vi "Main.vi"(8 "error in":errorcluster, 11 "Maestro Acq in":refnum<class "Maestro Acq.lvclass">) -> (0 "error out":errorcluster, 3 "Maestro Acq out":refnum<class "Maestro Acq.lvclass">)   [LabVIEW 2021, in "Maestro Acq.lvclass"]
doc: "The Queued Message Handler of a Worker."
uses:
  Maestro Acq.lvclass
  C:/Program Files (x86)/National Instruments/LabVIEW 2021/vi.lib/addons/_Workers/Library/Classes/Worker/Worker.lvclass
  Acquisition State.ctl
  Initialization Data.ctl
  <vilib>/addons/_Workers/Library/Classes/Message Queue/Message Queue.lvclass
  Hardware Maestro Config.ctl
  Maestro Acq.lvclass/Maestro Acq.ctl
  <vilib>/addons/_Workers/Library/Classes/Message/Enqueue Message to Self v2 - Silent Mode.vi
  <vilib>/addons/_Workers/Library/Classes/Message/Enqueue Message to Self v2.vi
  <vilib>/addons/_Workers/Library/Classes/Message/Enqueue Message to Queue.vi
  <vilib>/addons/_Workers/Library/Classes/Message/Message.lvclass
  Maestro Control/Maestro Control.lvclass
  C:/Program Files (x86)/National Instruments/LabVIEW 2021/vi.lib/addons/_Workers/Library/Classes/Workers Object/Workers Object.lvclass
  C:/Users/flepetit/Desktop/Gentec-maestro-Labview/Workers/Maestro Acq/Maestro Acq.lvclass
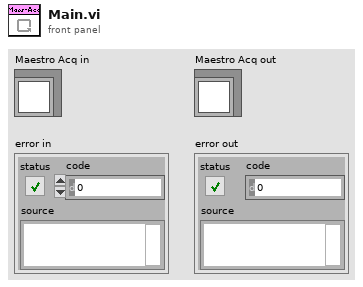
[diagram p1: front panel]
types:
  T1 = typedef "Maestro Acq.lvclass/Initialization Data.ctl" = cluster{"String":string, "Maestro Ctrl Queue":refnum<class "Message Queue.lvclass">, "Hardware Maestro Config":T2}
  T2 = typedef "Maestro Acq.lvclass/Hardware Maestro Config.ctl" = cluster{"Adress(ip)":string, "Port":i16}
  T3 = typedef "Maestro Acq.lvclass/Acquisition State.ctl" = enum16{"Idle", "Acquiring"}
  T4 = typedef "Workers.lvlib/Case Label.ctl" = string
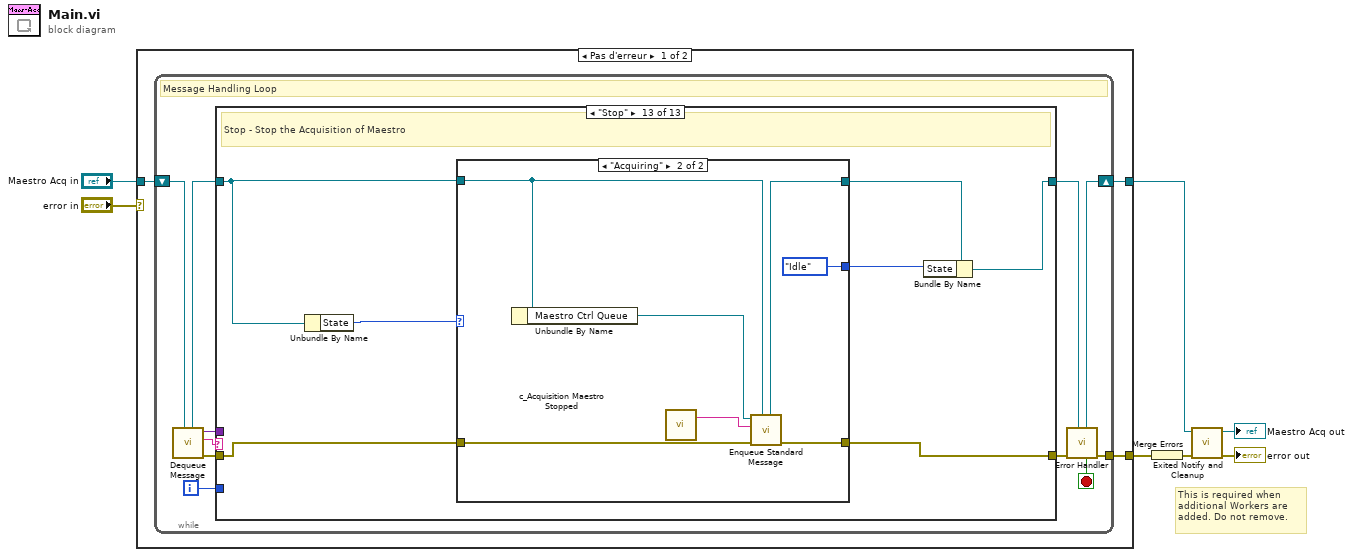
[diagram p0: block diagram]
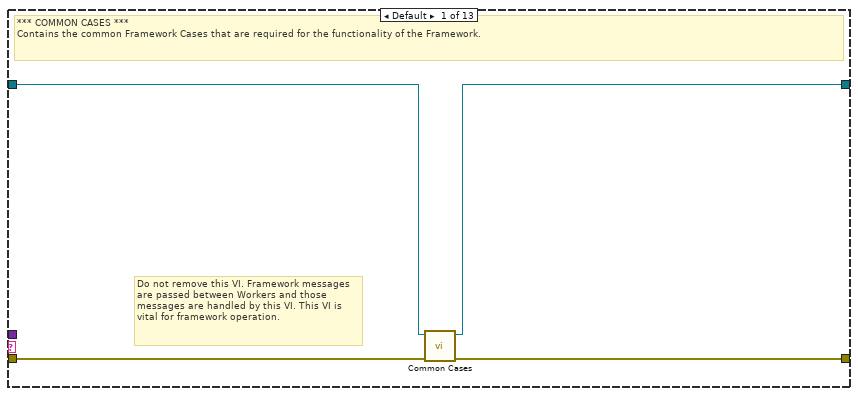
[diagram p2: hidden frame]
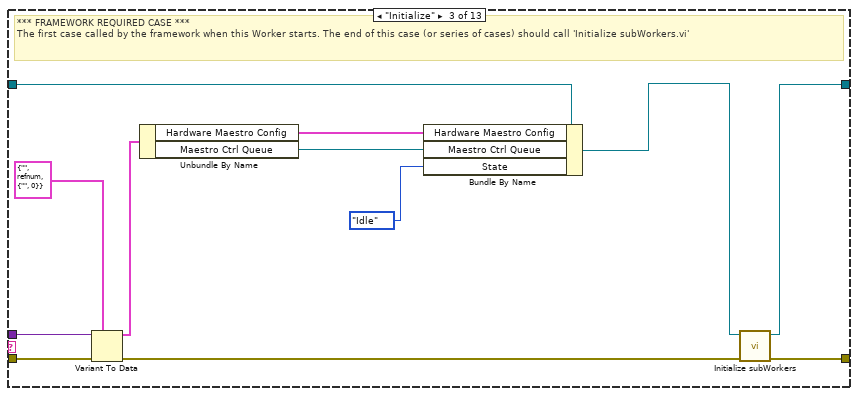
[diagram p4: hidden frame]
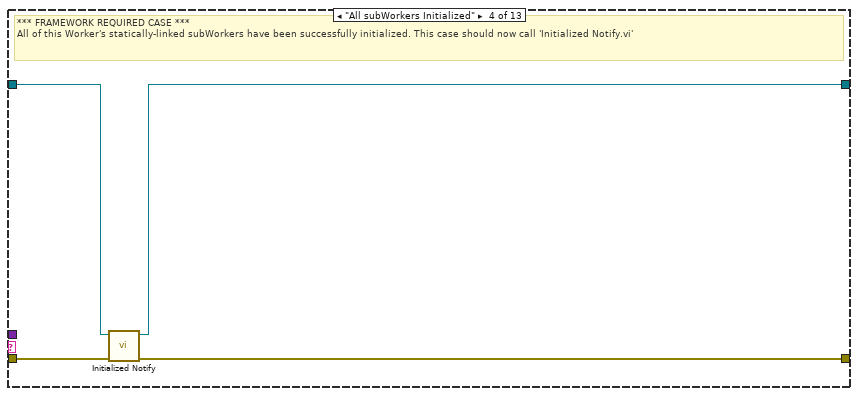
[diagram p5: hidden frame]
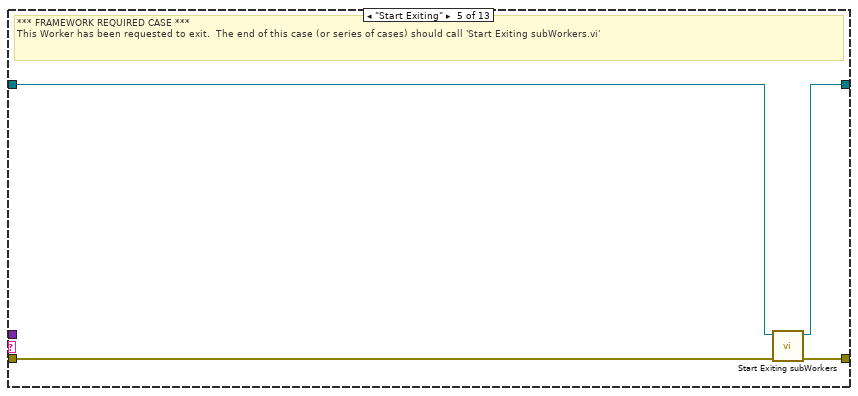
[diagram p6: hidden frame]
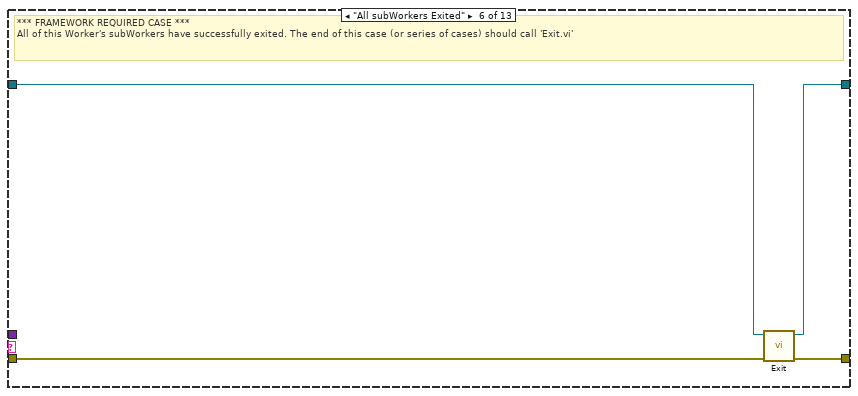
[diagram p7: hidden frame]
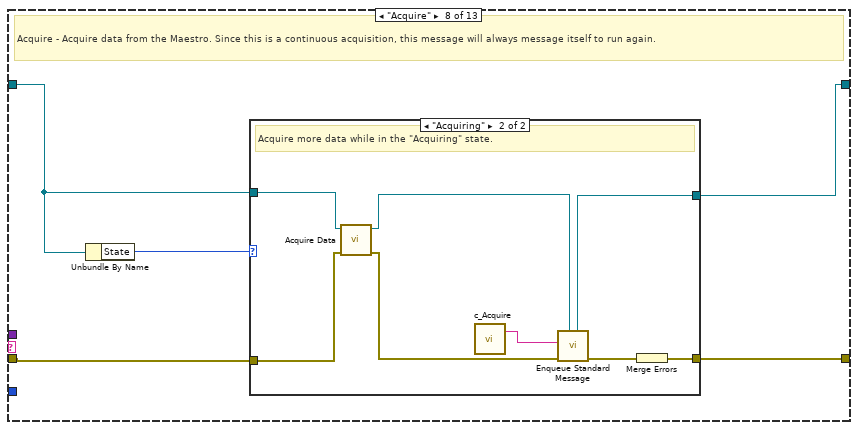
[diagram p9: hidden frame]
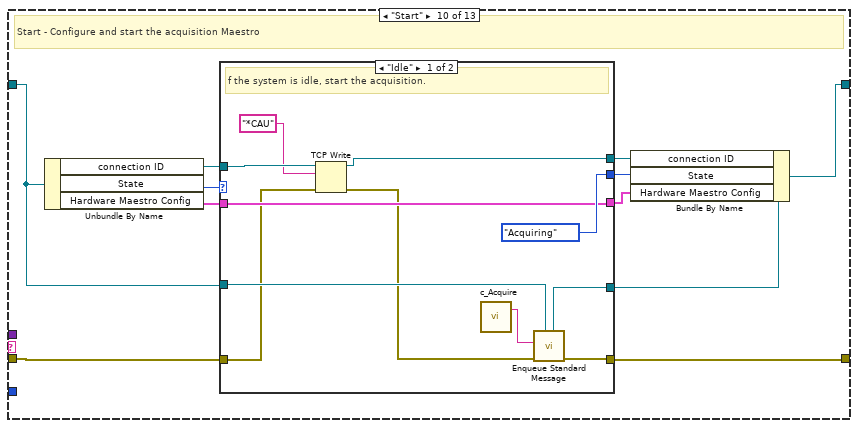
[diagram p12: hidden frame]
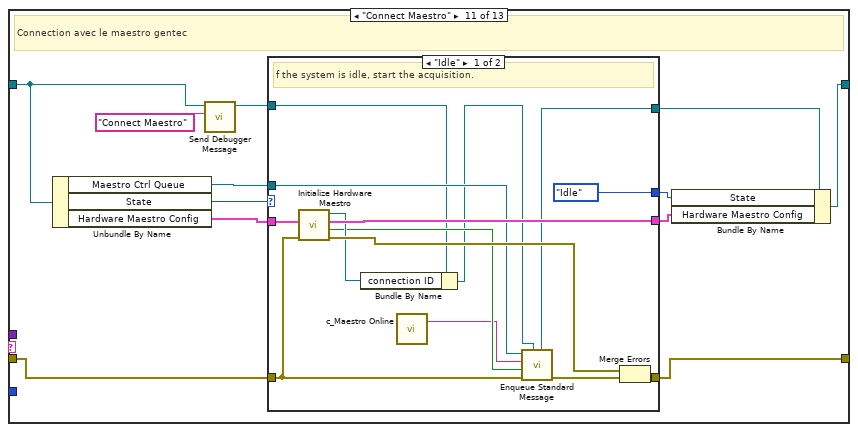
[diagram p14: hidden frame]
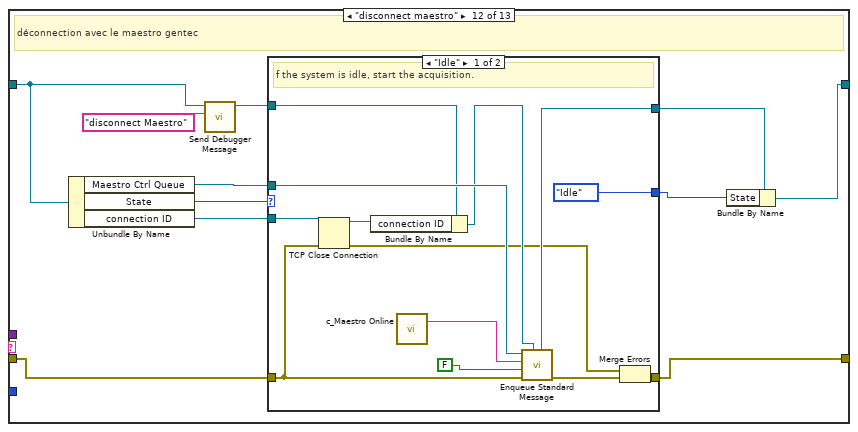
[diagram p16: hidden frame]
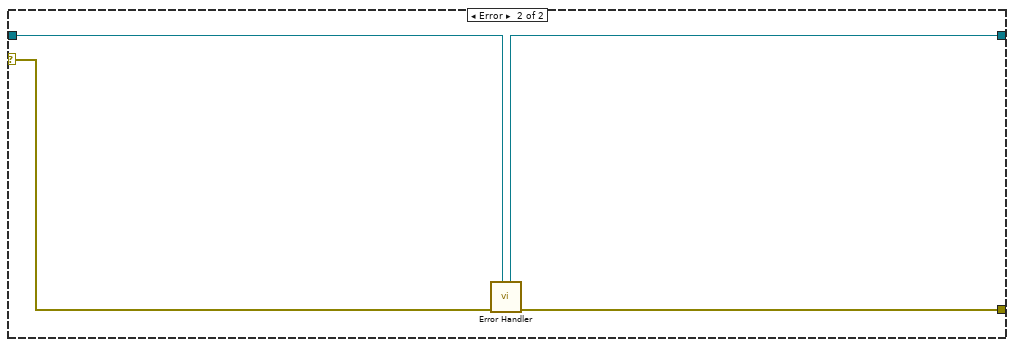
[diagram p19: hidden frame]
diagram:
  # "This is required when additional Workers are added. Do not remove."
  n1 = case shown="Pas d'erreur" "error in" {
    tunnel: "Maestro Acq in" -> [w8 w173]
    tunnel: [w10 w174] -> w6
    tunnel: [w9 w172] -> w7
    selector: "error in" -> [_ w175]
    frame No Error {
      n2 = while {
        shift-right: [w19] -> w9
        shift-left: w8 -> [w21]
        tunnel: [w20] -> w10
        i -> [w11]
        stop <- w12 stop-if-true
        # "Message Handling Loop"
        n3 = call-dynamic "Dequeue Message.vi"("Worker"=w21) -> ("error out"=w18:errorcluster, "Case out"=w13:string, "Data out"=w14:variant, "Worker out"=w16:refnum<class "Maestro Acq.lvclass">)  [unwired: 6 in, 1 out]
        n4 = case "Worker MHL Case Structure (DO NOT CHANGE LABEL NAME)" shown="\"Stop\"" w13 {
          tunnel: w18 -> [w25 w26 w37 w43 w44 w51 w52 w57 w70 w80 w103 w133 w159]
          tunnel: [w24 w26 w39 w42 w47 w50 w52 w56 w70 w81 w102 w132 w158] -> w17
          tunnel: w16 -> [w23 w27 w33 w41 w45 w49 w53 w54 w69 w79 w108 w137 w160]
          tunnel: [w22 w27 w38 w40 w46 w48 w53 w55 w69 w71 w98 w129 w155] -> w15
          tunnel: w14 -> [_ _ w35 _ _ _ _ _ _ _ _ _ _]
          tunnel: w11 -> [_ _ _ _ _ _ _ _ _ _ _ _ _]
          frame Default {
            # "Do not remove this VI. Framework messages are passed between Workers and those messages are handled by this VI. This VI is vital for framework operation."
            # "*** COMMON CASES ***\nContains the common Framework Cases that are required for the functionality of the Framework."
            n5 = call-dynamic "Common Cases.vi"("error in"=w25, "Worker in"=w23) -> ("error out"=w24:errorcluster, "Worker out"=w22:refnum<class "Maestro Acq.lvclass">)  [unwired: 8 in]
          }
          frame "------ FRAMEWORK REQUIRED CASES ------" {
            # "Start of Framework Required Cases"
          }
          frame "Initialize" {
            # "*** FRAMEWORK REQUIRED CASE ***\nThe first case called by the framework when this Worker starts. The end of this case (or series of cases) should call 'Initialize subWorkers.vi'"
            n6 = Variant To Data(error in=w37, type=T1 {"String"="", "Maestro Ctrl Queue"=refnum, "Hardware Maestro Config"={"Adress(ip)"="", "Port"=0}} ("Initialization Data"), Variant=w35) -> (data=w34:T1, error out=w36:errorcluster)
            n7 = Unbundle By Name(w34) -> ("Hardware Maestro Config"=w30:T2, "Maestro Ctrl Queue"=w28:refnum<class "Message Queue.lvclass">)
            n8 = Bundle By Name(cluster=w33, "Hardware Maestro Config"=w30, "Maestro Ctrl Queue"=w28, "State"=Acquisition_State."Idle") -> (w32:refnum<class "Maestro Acq.lvclass">)
            n9 = call-dynamic "Initialize subWorkers.vi"("error in"=w36, "Worker"=w32) -> ("error out"=w39:errorcluster, "dup Worker out"=w38:refnum<class "Maestro Acq.lvclass">)  [unwired: 8 in]
          }
          frame "All subWorkers Initialized" {
            # "*** FRAMEWORK REQUIRED CASE ***\nAll of this Worker's statically-linked subWorkers have been successfully initialized. This case should now call 'Initialized Notify.vi'"
            n10 = call-dynamic "Initialized Notify.vi"("error in"=w43, "Worker"=w41) -> ("error out"=w42:errorcluster, "dup Worker out"=w40:refnum<class "Maestro Acq.lvclass">)  [unwired: 8 in]
          }
          frame "Start Exiting" {
            # "*** FRAMEWORK REQUIRED CASE ***\nThis Worker has been requested to exit.  The end of this case (or series of cases) should call 'Start Exiting subWorkers.vi'"
            n11 = call-dynamic "Start Exiting subWorkers.vi"("error_in"=w44, "Worker"=w45) -> ("error out"=w47:errorcluster, "dup Worker out"=w46:refnum<class "Maestro Acq.lvclass">)  [unwired: 8 in]
          }
          frame "All subWorkers Exited" {
            # "*** FRAMEWORK REQUIRED CASE ***\nAll of this Worker's subWorkers have successfully exited. The end of this case (or series of cases) should call 'Exit.vi'"
            n12 = call-dynamic "Exit.vi"("error_in"=w51, "Worker"=w49) -> ("error out"=w50:errorcluster, "dup Worker out"=w48:refnum<class "Maestro Acq.lvclass">)  [unwired: 8 in]
          }
          frame "--------------Himself--------------" {
            # "End of Framework Required Cases"
          }
          frame "Acquire" {
            # "Acquire - Acquire data from the Maestro. Since this is a continuous acquisition, this message will always message itself to run again."
            n13 = Unbundle By Name(w54) -> ("State"=w58:T3)
            n14 = case shown="\"Acquiring\"" w58 {
              tunnel: w57 -> [w59 w64]
              tunnel: [w59 w67] -> w56
              tunnel: [w60 w66] -> w55
              tunnel: w54 -> [w60 w62]
              frame "Idle" {
                # "gnore \"Acquire\" messages when the acquisition is idle."
              }
              frame "Acquiring" {
                # "Acquire more data while in the \"Acquiring\" state."
                n15 = call "Acquire Data.vi"("error in (no error)"=w64, "Maestro Acq en entrée"=w62) -> ("error out"=w63:errorcluster, "Maestro Acq en sortie"=w61:refnum<class "Maestro Acq.lvclass">)  [unwired: 8 in]
                n16 = call "c_Acquire.vi"() -> ("Case Label"=w65:T4)  [unwired: 1 in]
                n17 = call-poly <vilib>:"Enqueue Standard Message.vi"("Worker"=w61, "error in"=w63, "Case Label"=w65) -> ("error out"=w68:errorcluster, "dup Worker out"=w66:refnum<class "Maestro Acq.lvclass">)  [unwired: 7 in]
                n18 = Merge Errors(w68) -> (w67:errorcluster)
              }
            }
          }
          frame "--------------From Maestro Control-----------------" {
          }
          frame "Start" {
            # "Start - Configure and start the acquisition Maestro"
            n19 = Unbundle By Name(w79) -> ("connection ID"=w75:refnum<k5>, "State"=w78:T3, "Hardware Maestro Config"=w77:T2)
            n20 = case shown="\"Idle\"" w78 {
              selector: w78 -> [_ w95]
              tunnel: [w89 w97] -> w73
              tunnel: w79 -> [w88 w97]
              tunnel: [w85 w96] -> w81
              tunnel: w80 -> [w86 w96]
              tunnel: [Acquisition_State."Acquiring" ("Acquisition State") w95] -> w72
              tunnel: w77 -> [w90 w94]
              tunnel: [w90 w94] -> w76
              tunnel: w75 -> [w87 w93]
              tunnel: [w83 w93] -> w74
              frame "Idle" {
                # "f the system is idle, start the acquisition."
                n21 = TCP Write(connection ID=w87, data in="*CAU" ("string"), error in (no error)=w86) -> (connection ID out=w83:refnum<k5>, error out=w82:errorcluster)  [unwired: 1 in, 1 out]
                n22 = call "c_Acquire.vi"() -> ("Case Label"=w91:T4)  [unwired: 1 in]
                n23 = call-poly <vilib>:"Enqueue Standard Message.vi"("Worker"=w88, "error in"=w82, "Case Label"=w91) -> ("error out"=w85:errorcluster, "dup Worker out"=w89:refnum<class "Maestro Acq.lvclass">)  [unwired: 7 in]
              }
              frame "Acquiring" {
                # "The system is already acquiring. Ignore the \"Start\" message."
              }
            }
            n24 = Bundle By Name(cluster=w73, "connection ID"=w74, "State"=w72, "Hardware Maestro Config"=w76) -> (w71:refnum<class "Maestro Acq.lvclass">)
          }
          frame "Connect Maestro" {
            # "Connection avec le maestro gentec"
            n25 = Unbundle By Name(w108) -> ("Maestro Ctrl Queue"=w107:refnum<class "Message Queue.lvclass">, "State"=w106:T3, "Hardware Maestro Config"=w105:T2)
            n26 = call-dynamic "Send Debugger Message.vi"("Message String"="Connect Maestro", "Worker"=w108) -> ("dup Worker out"=w104:refnum<class "Maestro Acq.lvclass">)  [unwired: 8 in, 1 out]
            n27 = case shown="\"Idle\"" w106 {
              selector: w106 -> [_ w126]
              tunnel: [w116 w124] -> w99
              tunnel: [w123 w127] -> w102
              tunnel: w103 -> [w121 w127]
              tunnel: [Acquisition_State."Idle" ("Acquisition State") w126] -> w101
              tunnel: w105 -> [w119 w125]
              tunnel: [w118 w125] -> w100
              tunnel: w107 -> [w113 _]
              tunnel: w104 -> [w111 w124]
              frame "Idle" {
                # "f the system is idle, start the acquisition."
                n28 = call "Initialize Hardware Maestro.vi"("error in (no error)"=w121, "Hardware Maestro Config"=w119) -> ("error out"=w120:errorcluster, "Maestro Online"=w114:bool, "Hardware Maestro Config 2"=w118:T2, "connection ID"=w115:refnum<k5>)  [unwired: 6 in]
                n29 = Bundle By Name(cluster=w111, "connection ID"=w115) -> (w110:refnum<class "Maestro Acq.lvclass">)
                n30 = call "c_Maestro Online.vi"() -> ("Case Label"=w112:T4)  [unwired: 1 in]
                n31 = call-poly <vilib>:"Enqueue Standard Message.vi"("Worker"=w110, "error in"=w121, "Data"=w114, "Case Label"=w112, "Message Queue"=w113) -> ("error out"=w117:errorcluster, "dup Worker out"=w116:refnum<class "Maestro Acq.lvclass">)  [unwired: 4 in, 1 out]
                n32 = Merge Errors(w120, w117) -> (w123:errorcluster)
              }
              frame "Acquiring" {
                # "The system is already acquiring. Ignore the \"Start\" message."
              }
            }
            n33 = Bundle By Name(cluster=w99, "State"=w101, "Hardware Maestro Config"=w100) -> (w98:refnum<class "Maestro Acq.lvclass">)
          }
          frame "disconnect maestro" {
            # "déconnection avec le maestro gentec"
            n34 = Unbundle By Name(w137) -> ("Maestro Ctrl Queue"=w136:refnum<class "Message Queue.lvclass">, "State"=w135:T3, "connection ID"=w128:refnum<k5>)
            n35 = call-dynamic "Send Debugger Message.vi"("Message String"="disconnect Maestro", "Worker"=w137) -> ("dup Worker out"=w134:refnum<class "Maestro Acq.lvclass">)  [unwired: 8 in, 1 out]
            n36 = case shown="\"Idle\"" w135 {
              selector: w135 -> [_ w153]
              tunnel: [w148 w152] -> w130
              tunnel: [w151 w154] -> w132
              tunnel: w133 -> [w142 w154]
              tunnel: [Acquisition_State."Idle" ("Acquisition State") w153] -> w131
              tunnel: w136 -> [w147 _]
              tunnel: w134 -> [w145 w152]
              tunnel: w128 -> [w143 _]
              frame "Idle" {
                # "f the system is idle, start the acquisition."
                n37 = TCP Close Connection(connection ID=w143, error in (no error)=w142) -> (connection ID out=w140:refnum<k5>, error out=w141:errorcluster)  [unwired: 1 in]
                n38 = Bundle By Name(cluster=w145, "connection ID"=w140) -> (w144:refnum<class "Maestro Acq.lvclass">)
                n39 = call "c_Maestro Online.vi"() -> ("Case Label"=w146:T4)  [unwired: 1 in]
                n40 = call-poly <vilib>:"Enqueue Standard Message.vi"("Worker"=w144, "error in"=w142, "Data"=FALSE, "Case Label"=w146, "Message Queue"=w147) -> ("error out"=w149:errorcluster, "dup Worker out"=w148:refnum<class "Maestro Acq.lvclass">)  [unwired: 4 in, 1 out]
                n41 = Merge Errors(w141, w149) -> (w151:errorcluster)
              }
              frame "Acquiring" {
                # "The system is already acquiring. Ignore the \"Start\" message."
              }
            }
            n42 = Bundle By Name(cluster=w130, "State"=w131) -> (w129:refnum<class "Maestro Acq.lvclass">)
          }
          frame "Stop" {
            # "Stop - Stop the Acquisition of Maestro"
            n43 = Unbundle By Name(w160) -> ("State"=w161:T3)
            n44 = case shown="\"Acquiring\"" w161 {
              selector: w161 -> [w162 _]
              tunnel: w160 -> [w164 w166]
              tunnel: [w164 w171] -> w156
              tunnel: w159 -> [w163 w170]
              tunnel: [w163 w169] -> w158
              tunnel: [w162 Acquisition_State."Idle" ("State")] -> w157
              frame "Idle", Default {
              }
              frame "Acquiring" {
                n45 = Unbundle By Name(w166) -> ("Maestro Ctrl Queue"=w165:refnum<class "Message Queue.lvclass">)
                n46 = call "c_Acquisition Maestro Stopped.vi"() -> ("Case Label"=w167:T4)  [unwired: 1 in]
                n47 = call-poly <vilib>:"Enqueue Standard Message.vi"("Worker"=w166, "error in"=w170, "Case Label"=w167, "Message Queue"=w165) -> ("error out"=w169:errorcluster, "dup Worker out"=w171:refnum<class "Maestro Acq.lvclass">)  [unwired: 5 in, 1 out]
              }
            }
            n48 = Bundle By Name(cluster=w156, "State"=w157) -> (w155:refnum<class "Maestro Acq.lvclass">)
          }
        }
        n49 = call-dynamic "Error Handler.vi"("Worker"=w15, "error_in"=w17) -> ("error out"=w20:errorcluster, "Stop Loop"=w12:bool, "Worker out"=w19:refnum<class "Maestro Acq.lvclass">)  [unwired: 7 in]
      }
    }
    frame Error {
      n50 = call-dynamic "Error Handler.vi"("Worker"=w173, "error_in"=w175) -> ("error out"=w174:errorcluster, "Worker out"=w172:refnum<class "Maestro Acq.lvclass">)  [unwired: 7 in, 1 out]
    }
  }
  n51 = Merge Errors(w6) -> (w3:errorcluster)
  n52 = call-dynamic "Exited Notify and Cleanup.vi"("error_in"=w3, "Worker"=w7) -> ("error out"=→"error out":errorcluster, "dup Worker out"=→"Maestro Acq out":refnum<class "Maestro Acq.lvclass">)  [unwired: 8 in]
